vi "DSF.Engine.Plugin.Get Plugin Configuration.vi"(8 "error in (no error)":errorcluster, 11 "Plugin in":refnum<class "Plugin.lvclass">) -> (0 "error out":errorcluster, 2 "Plugin Configuration":refnum<class "DSF.Shared.Configuration.Plugin.lvclass">, 3 "Plugin out":refnum<class "Plugin.lvclass">)   [LabVIEW 2016, in "DSF.Engine.lvlib" / "Plugin.lvclass"]
uses:
  Plugin.lvclass
  Shared/Classes/Plugin/DSF.Shared.Configuration.Plugin.lvclass
  Plugin.lvclass/Plugin.ctl
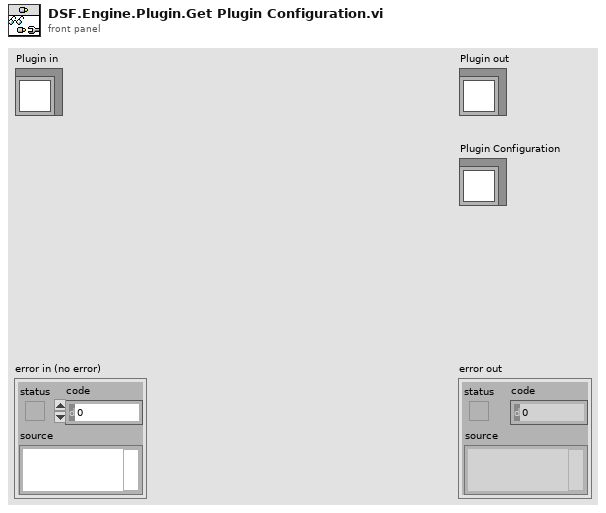
[diagram p1: front panel]
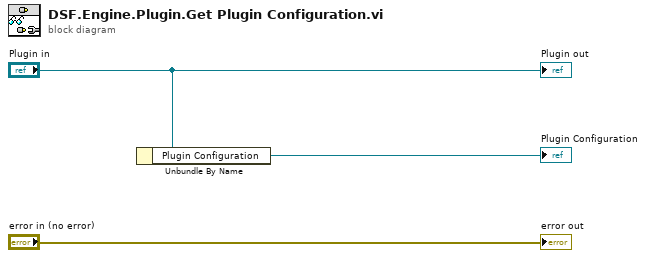
[diagram p0: block diagram]
diagram:
  n1 = Unbundle By Name("Plugin in") -> ("Plugin Configuration"=→"Plugin Configuration":refnum<class "DSF.Shared.Configuration.Plugin.lvclass">)
  "error out" <- "error in (no error)"
  "Plugin out" <- "Plugin in"
